vi "NI_FPGA_PPG.get library version.vi"() -> (0 "nameAndVersion":string)   [LabVIEW 2014, in "NI_FPGA_PPG.lvlib"]
doc: "obtain name and version of a library as a string"
uses:
  NI_FPGA_PPG.lvlib
  CSlibraries/UtilityLib/UtilityLib.lvlib
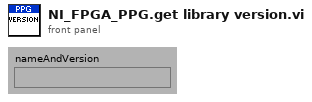
[diagram p1: front panel]
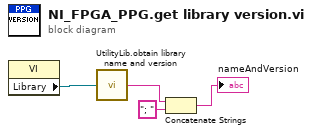
[diagram p0: block diagram]
diagram:
  n1 = property class="VI"() -> ("Library"=w4:refnum<vi>)  [unwired: 2 in, 2 out]
  n2 = call "UtilityLib.obtain library name and version.vi"("Library"=w4) -> ("nameAndVersion"=w3:string)
  n3 = Concatenate Strings(w3, "; " ("element")) -> (→"nameAndVersion":string)
